vi "GetScopeData.vi"(8 "error in (no error)":errorcluster, 10 "number of points":i32=2000 min=1 step=1, 11 "controller in":refnum<k24>) -> (0 "error out":errorcluster, 2 "scope data":T1, 3 "controller out":refnum<k24>)   [LabVIEW 2010]
uses:
  c:/aerotech/controller/5.xx.xxx/ensemble/pc/labview/2010/bin/Aerotech.Ensemble.dll
  bin/Aerotech.Ensemble.dll
  AxisDataResults.ctl
  ControllerDataResults.ctl
  c:/aerotech/controller/5.xx.xxx/ensemble/pc/labview/2010/bin/Aerotech.Ensemble.LabVIEW.dll
  bin/Aerotech.Ensemble.LabVIEW.dll
panel:
  in  "ControllerDataResults Type":T1
  in  "AxisDataResults Type":T2
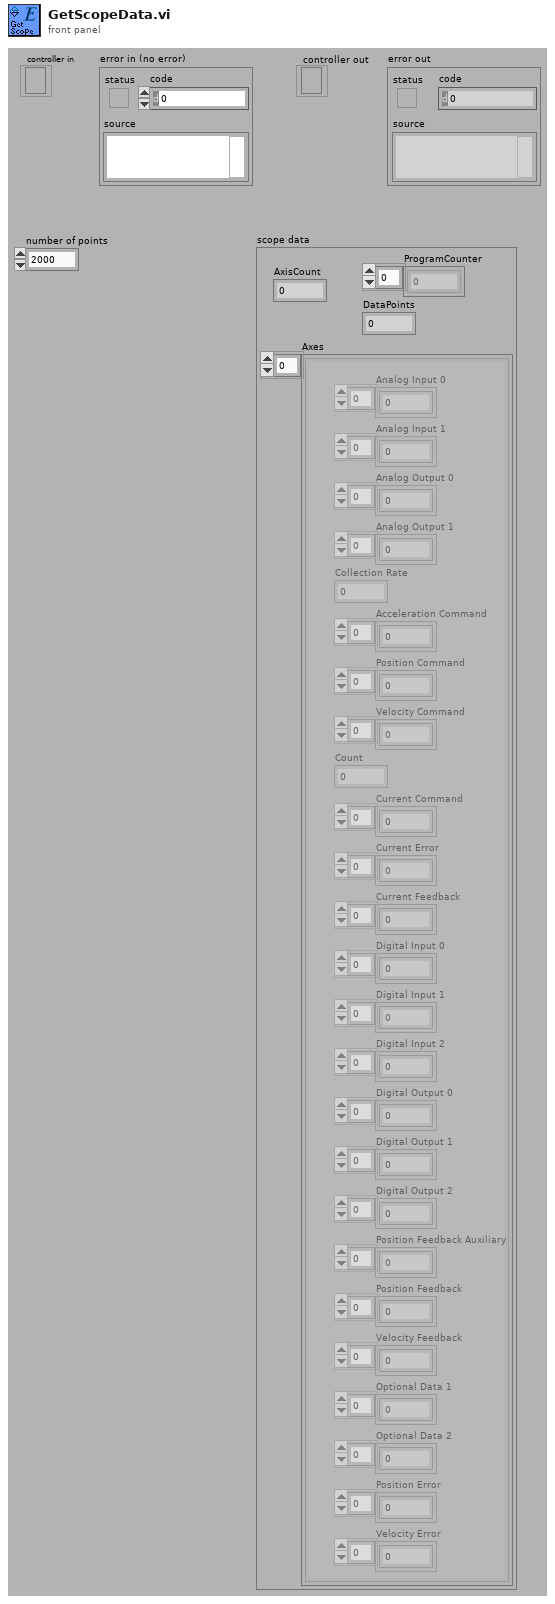
[diagram p1: front panel]
types:
  T1 = typedef "ControllerDataResults.ctl" = cluster{"AxisCount":i32, "DataPoints":i32, "ProgramCounter":i32[], "Axes":T2[]}
  T2 = typedef "AxisDataResults.ctl" = cluster{"Analog Input 0":dbl[], "Analog Input 1":dbl[], "Analog Output 0":dbl[], "Analog Output 1":dbl[], "Collection Rate":dbl, "Acceleration Command":dbl[], "Position Command":dbl[], "Velocity Command":dbl[], "Count":i32, "Current Command":sgl[], "Current Error":sgl[], "Current Feedback":sgl[], "Digital Input 0":i32[], "Digital Input 1":i32[], "Digital Input 2":i32[], "Digital Output 0":i32[], "Digital Output 1":i32[], "Digital Output 2":i32[], "Position Feedback Auxiliary":dbl[], "Position Feedback":dbl[], "Velocity Feedback":dbl[], "Optional Data 1":dbl[], "Optional Data 2":dbl[], "Position Error":dbl[], "Velocity Error":dbl[]}
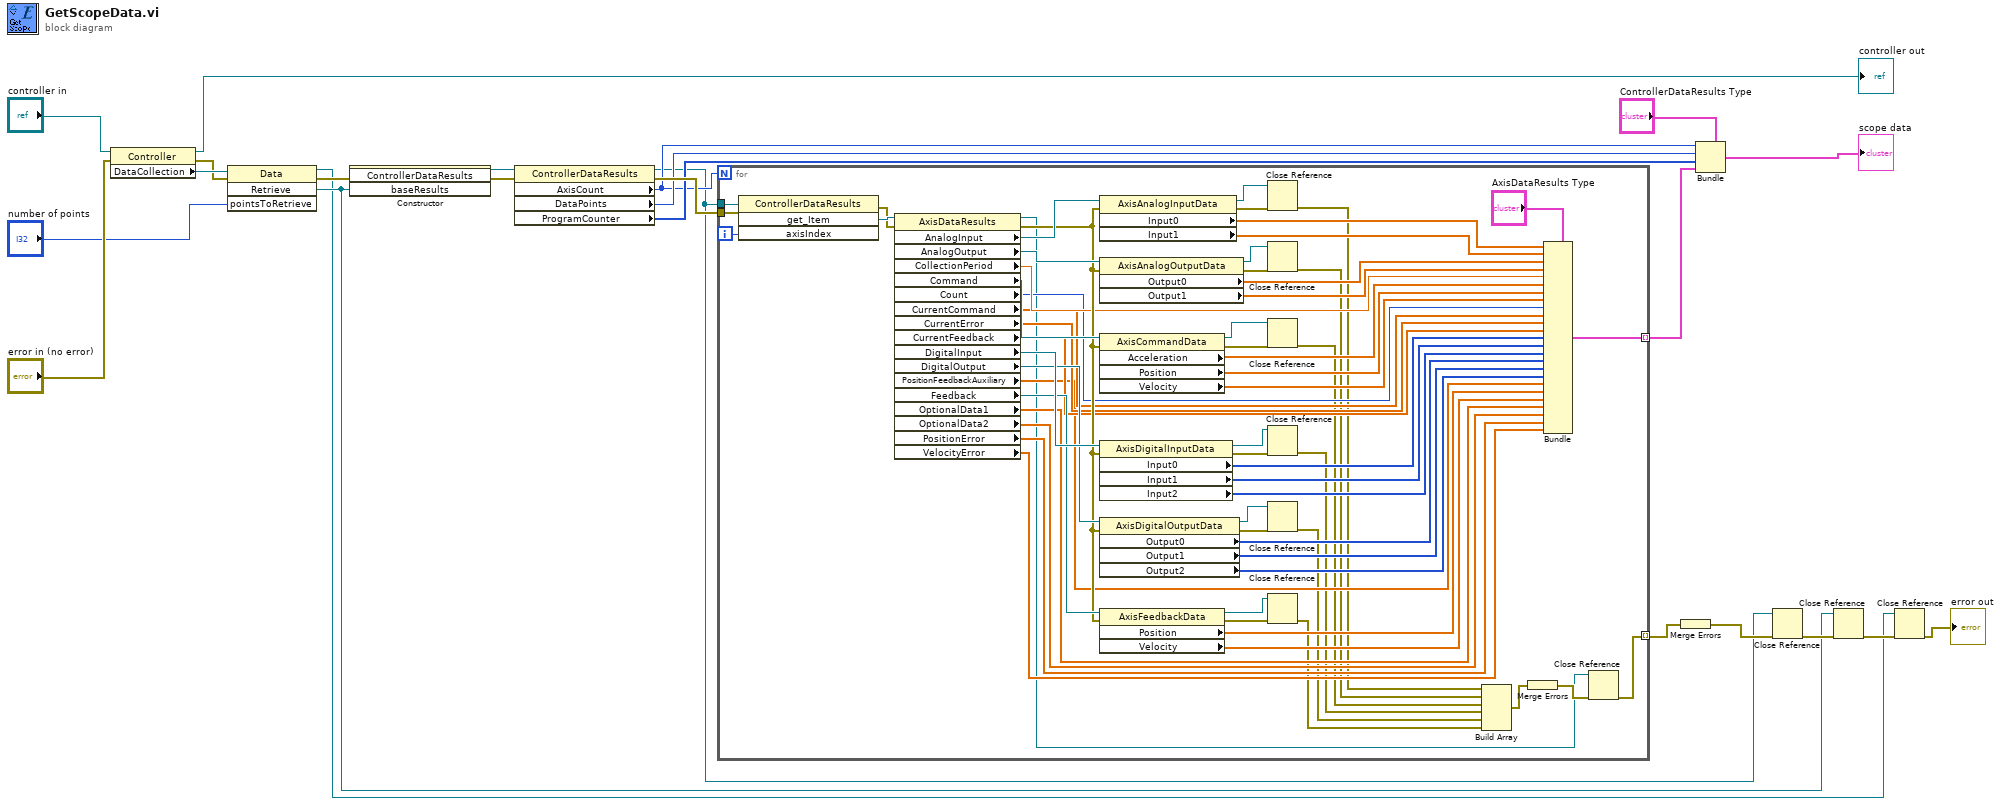
[diagram p0: block diagram]
diagram:
  n1 = property class="Controller"(reference="controller in", error in="error in (no error)") -> (reference out=→"controller out":refnum<k24>, error out=w21:errorcluster, "DataCollection"=w22:refnum<k24>)
  n2 = invoke class="Data" method="Retrieve"(reference=w22, error in=w21, "pointsToRetrieve"="number of points") -> (reference out=w1:refnum<k24>, error out=w8:errorcluster, "Retrieve"=w2:refnum<k24>)  [unwired: 1 in, 1 out]
  n3 = constructor class="ControllerDataResults"(error in=w8, "baseResults"=w2) -> (reference out=w9:refnum<k24>, error out=w10:errorcluster)  [unwired: 2 in, 2 out]
  n4 = property class="ControllerDataResults"(reference=w9, error in=w10) -> (reference out=w6:refnum<k24>, error out=w15:errorcluster, "AxisCount"=w11:i32, "DataPoints"=w13:i32, "ProgramCounter"=w12:i32[])
  n5 = for {
    N: w11 -> [_]
    tunnel: w6 -> [w85]
    tunnel: w15 -> [w84]
    tunnel: [w71] -> w14 mode=indexing
    tunnel: [w26] -> w16 mode=indexing
    i -> [w83]
    n6 = invoke class="ControllerDataResults" method="get_Item"(reference=w85, error in=w84, "axisIndex"=w83) -> (error out=w81:errorcluster, "get_Item"=w82:refnum<k24>)  [unwired: 1 in, 2 out]
    n7 = property class="AxisDataResults"(reference=w82, error in=w81) -> (reference out=w25:refnum<k24>, error out=w74:errorcluster, "AnalogInput"=w80:refnum<k24>, "AnalogOutput"=w79:refnum<k24>, "CollectionPeriod"=w65:dbl, "Command"=w78:refnum<k24>, "Count"=w64:i32, "CurrentCommand"=w63:sgl[], "CurrentError"=w62:sgl[], "CurrentFeedback"=w61:sgl[], "DigitalInput"=w77:refnum<k24>, "DigitalOutput"=w76:refnum<k24>, "PositionFeedbackAuxiliary"=w54:dbl[], "Feedback"=w75:refnum<k24>, "OptionalData1"=w51:dbl[], "OptionalData2"=w50:dbl[], "PositionError"=w49:dbl[], "VelocityError"=w48:dbl[])
    n8 = property class="AxisAnalogInputData"(reference=w80, error in=w74) -> (reference out=w43:refnum<k24>, error out=w44:errorcluster, "Input0"=w73:dbl[], "Input1"=w72:dbl[])
    n9 = property class="AxisAnalogOutputData"(reference=w79, error in=w74) -> (reference out=w40:refnum<k24>, error out=w42:errorcluster, "Output0"=w70:dbl[], "Output1"=w69:dbl[])
    n10 = property class="AxisCommandData"(reference=w78, error in=w74) -> (reference out=w37:refnum<k24>, error out=w38:errorcluster, "Acceleration"=w68:dbl[], "Position"=w67:dbl[], "Velocity"=w66:dbl[])
    n11 = property class="AxisDigitalInputData"(reference=w77, error in=w74) -> (reference out=w29:refnum<k24>, error out=w28:errorcluster, "Input0"=w60:i32[], "Input1"=w59:i32[], "Input2"=w58:i32[])
    n12 = property class="AxisDigitalOutputData"(reference=w76, error in=w74) -> (reference out=w34:refnum<k24>, error out=w36:errorcluster, "Output0"=w57:i32[], "Output1"=w56:i32[], "Output2"=w55:i32[])
    n13 = property class="AxisFeedbackData"(reference=w75, error in=w74) -> (reference out=w30:refnum<k24>, error out=w31:errorcluster, "Position"=w53:dbl[], "Velocity"=w52:dbl[])
    n14 = Close Reference(reference=w43, error in (no error)=w44) -> (error out=w45:errorcluster)
    n15 = Close Reference(reference=w40, error in (no error)=w42) -> (error out=w41:errorcluster)
    n16 = Close Reference(reference=w37, error in (no error)=w38) -> (error out=w39:errorcluster)
    n17 = Close Reference(reference=w29, error in (no error)=w28) -> (error out=w33:errorcluster)
    n18 = Close Reference(reference=w34, error in (no error)=w36) -> (error out=w35:errorcluster)
    n19 = Close Reference(reference=w30, error in (no error)=w31) -> (error out=w32:errorcluster)
    n20 = Build Array(w45, w41, w39, w33, w35, w32) -> (w46:errorcluster[])
    n21 = Merge Errors(w46) -> (w27:errorcluster)
    n22 = Bundle(cluster="AxisDataResults Type", "Analog Input 0"=w73, "Analog Input 1"=w72, "Analog Output 0"=w70, "Analog Output 1"=w69, "Collection Rate"=w65, "Acceleration Command"=w68, "Position Command"=w67, "Velocity Command"=w66, "Count"=w64, "Current Command"=w63, "Current Error"=w62, "Current Feedback"=w61, "Digital Input 0"=w60, "Digital Input 1"=w59, "Digital Input 2"=w58, "Digital Output 0"=w57, "Digital Output 1"=w56, "Digital Output 2"=w55, "Position Feedback Auxiliary"=w54, "Position Feedback"=w53, "Velocity Feedback"=w52, "Optional Data 1"=w51, "Optional Data 2"=w50, "Position Error"=w49, "Velocity Error"=w48) -> (w71:T2)
    n23 = Close Reference(reference=w25, error in (no error)=w27) -> (error out=w26:errorcluster)
  }
  n24 = Merge Errors(w16) -> (w7:errorcluster)
  n25 = Bundle(cluster="ControllerDataResults Type", "AxisCount"=w11, "DataPoints"=w13, "ProgramCounter"=w12, "Axes"=w14) -> (→"scope data":T1)
  n26 = Close Reference(reference=w6, error in (no error)=w7) -> (error out=w3:errorcluster)
  n27 = Close Reference(reference=w2, error in (no error)=w3) -> (error out=w4:errorcluster)
  n28 = Close Reference(reference=w1, error in (no error)=w4) -> (error out=→"error out":errorcluster)
